vi "writeToXML.vi"(8 "error in (no error)":errorcluster, 10 "Class Label":string="TCSIersStatus", 11 "TCSIersStatus in":refnum<class "TCSIersStatus.lvclass">) -> (0 "error out":errorcluster, 2 "XMLout":string="<TCSIersStatus>\n  <currentTimeActivity>Busy</currentTimeActivity>\n  <deltaAT>0</deltaAT>\n  <deltaUT>0</deltaUT>\n  <mjd>0</mjd>\n  <statusMessage/>\n  <timeActivityMessage/>\n  <timeHealthState>GOOD</timeHealthState>\n  <xpm>0</xpm>\n  <ypm>0</ypm>\n</TCSIersStatus>", 3 "TCSIersStatus out":refnum<class "TCSIersStatus.lvclass">)   [LabVIEW 2014, in "TCSDataDefinitions.lvlib" / "TCSTimeComponentStatus.lvlib" / "TCSIersStatus.lvclass"]
uses:
  TCSIersStatus.lvclass
  <userlib>/Common/UnitsAndXML/FlattenItemWithUnitToXML/FlattenTimeToXML/TimeUnit.ctl
  <userlib>/Common/UnitsAndXML/FlattenItemWithUnitToXML/FlattenPlaneAngleToXML/PlaneAngleUnit.ctl
  TCSIersStatus.lvclass/TCSIersStatus.ctl
  <userlib>/Common/UnitsAndXML/UnitsAndXML.lvlib
  <userlib>/Common/XML/XMLGenerator/XMLGenerator.lvclass
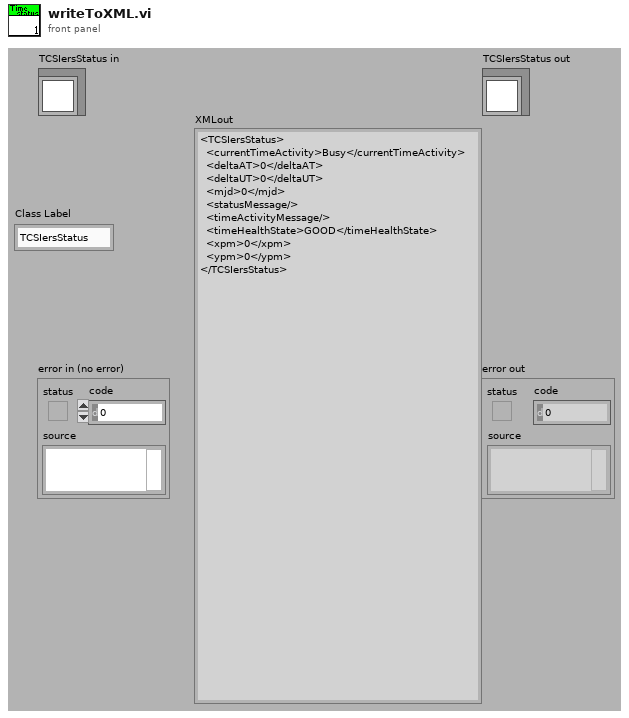
[diagram p1: front panel]
types:
  T1 = typedef "UnitsAndXML.lvlib/PlaneAngleUnit.ctl" = enum16{"rad", "deg", "'", "\""}
  T2 = typedef "UnitsAndXML.lvlib/TimeUnit.ctl" = enum16{"s", "d", "h", "min", "a"}
  T3 = typedef "TCSDataDefinitions.lvlib/TCSTimeComponentStatus.lvlib/ActivityValues.ctl" = enum16{"Busy", "Error", "Idle"}
  T4 = typedef "TCSDataDefinitions.lvlib/TCSPublicStatus.lvlib/TCSHealthValues.ctl" = enum16{"GOOD", "WARNING", "BAD"}
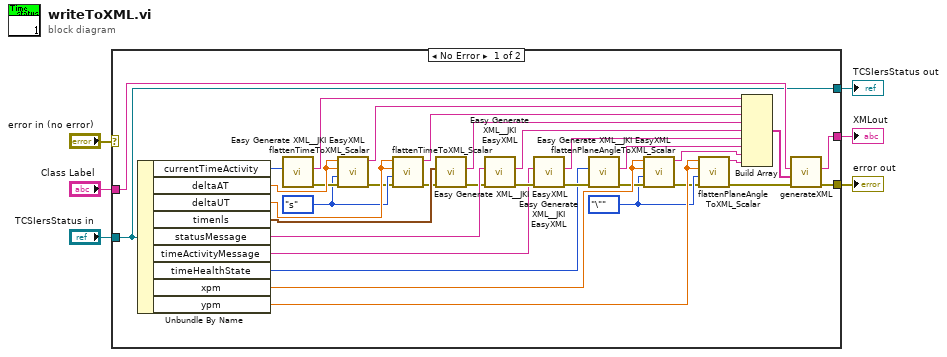
[diagram p0: block diagram]
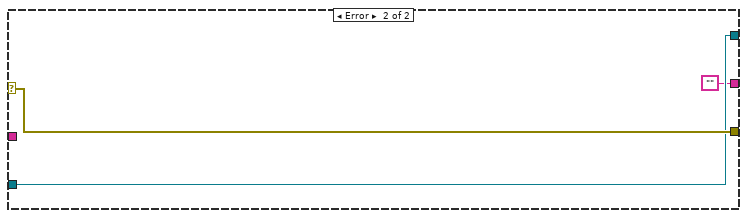
[diagram p2: hidden frame]
diagram:
  n1 = case shown="No Error" "error in (no error)" {
    selector: "error in (no error)" -> [_ w43]
    tunnel: [w13 w43] -> w5
    tunnel: [w11 w42] -> w3
    tunnel: "TCSIersStatus in" -> [w11 w42]
    tunnel: [w23 ""] -> w2
    tunnel: "Class Label" -> [w22 _]
    frame No Error {
      w17 = PlaneAngleUnit."\"" ("planeAngleUnitInXML")
      w29 = TimeUnit."s" ("timeUnitInXML")
      n2 = Unbundle By Name(w11) -> ("currentTimeActivity"=w38:T3, "deltaAT"=w34:dbl[unit], "deltaUT"=w30:dbl[unit], "timenls"=w10:timestamp, "statusMessage"=w37:string, "timeActivityMessage"=w36:string, "timeHealthState"=w35:T4, "xpm"=w20:dbl[unit], "ypm"=w18:dbl[unit])
      n3 = call <vilib>:"Easy Generate XML__JKI EasyXML.vi"("LabVIEW Data"=w38) -> ("error out"=w33:errorcluster, "XML String"=w32:string)  [unwired: 9 in]
      n4 = call <userlib>:"flattenTimeToXML_Scalar.vi"("error in (no error)"=w33, "timeUnitInXML"=w29, "timeAgain"=w34, "time"=w34) -> ("error out"=w28:errorcluster, "xmlString"=w31:string)  [unwired: 6 in]
      n5 = call <userlib>:"flattenTimeToXML_Scalar.vi"("error in (no error)"=w28, "timeUnitInXML"=w29, "timeAgain"=w30, "time"=w30) -> ("error out"=w8:errorcluster, "xmlString"=w27:string)  [unwired: 6 in]
      n6 = call <vilib>:"Easy Generate XML__JKI EasyXML.vi"("error in (no error)"=w8, "LabVIEW Data"=w10) -> ("error out"=w7:errorcluster, "XML String"=w9:string)  [unwired: 8 in]
      n7 = call <vilib>:"Easy Generate XML__JKI EasyXML.vi"("error in (no error)"=w7, "LabVIEW Data"=w37) -> ("error out"=w40:errorcluster, "XML String"=w26:string)  [unwired: 8 in]
      n8 = call <vilib>:"Easy Generate XML__JKI EasyXML.vi"("error in (no error)"=w40, "LabVIEW Data"=w36) -> ("error out"=w39:errorcluster, "XML String"=w25:string)  [unwired: 8 in]
      n9 = call <vilib>:"Easy Generate XML__JKI EasyXML.vi"("error in (no error)"=w39, "LabVIEW Data"=w35) -> ("error out"=w19:errorcluster, "XML String"=w21:string)  [unwired: 8 in]
      n10 = call <userlib>:"flattenPlaneAngleToXML_Scalar.vi"("error in (no error)"=w19, "planeAngleUnitInXML"=w17, "planeAngleAgain"=w20, "planeAngle"=w20) -> ("error out"=w15:errorcluster, "xmlString"=w12:string)  [unwired: 6 in]
      n11 = call <userlib>:"flattenPlaneAngleToXML_Scalar.vi"("error in (no error)"=w15, "planeAngleUnitInXML"=w17, "planeAngleAgain"=w18, "planeAngle"=w18) -> ("error out"=w14:errorcluster, "xmlString"=w16:string)  [unwired: 6 in]
      n12 = Build Array(w32, w31, w27, w9, w26, w25, w21, w12, w16) -> (w24:string[])
      n13 = call <userlib>:"generateXML.vi"("error in"=w14, "childrenXML"=w24, "elementName"=w22) -> ("error out"=w13:errorcluster, "XML out"=w23:string)  [unwired: 6 in, 1 out]
    }
    frame Error {
    }
  }
  "error out" <- w5
  "TCSIersStatus out" <- w3
  "XMLout" <- w2
